vi "Wrap TPCANMessageType.vi"(10 "TPCANMessageType Numeric":u8) -> (2 "TPCANMessageType out Strings":string, 3 "TPCANMessageType Numeric out":u8)   [LabVIEW 2016]
doc: "TPCANMessageType defines the Message type\nof a CAN message that should be send.\nIn the case of seinding a CAN message\nit can have the values below.\n\nPCAN Message Types:\nPCAN_MESSAGE_STANDARD 0x00\nPCAN_MESSAGE_RTR 0x01\nPCAN_MESSAGE_EXTENDED 0x02\nPCAN_MESSAGE_FD 0x04\nPCAN_MESSAGE_BRS 0x08\nPCAN_MESSAGE_ESI 0x10\nPCAN_MESSAGE_STATUS 0x80\n\nIn case of receiving messages from the\nPCAN driver is can look like the the list \nbefore but it also can be a bitfild.\nThat means that more than exact one\nreturn value within a single numeric is\npossible.\nTo make things more easy the VI is\ncapable to decode the PCAN drivers\nreturned value."
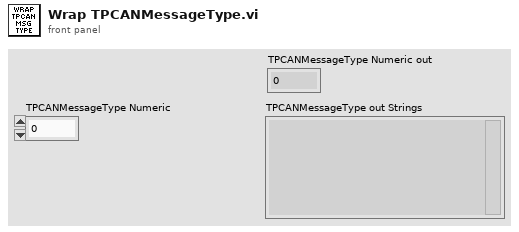
[diagram p1: front panel]
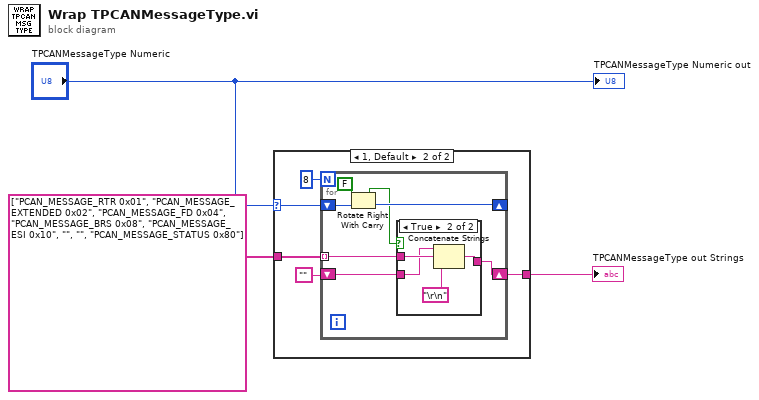
[diagram p0: block diagram]
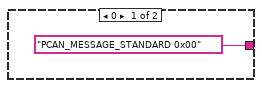
[diagram p2: hidden frame]
diagram:
  n1 = case shown="1, Default" "TPCANMessageType Numeric" {
    selector: "TPCANMessageType Numeric" -> [_ w5]
    tunnel: string[] ["PCAN_MESSAGE_RTR 0x01", "PCAN_MESSAGE_EXTENDED 0x02", "PCAN_MESSAGE_FD 0x04", "PCAN_MESSAGE_BRS 0x08", "PCAN_MESSAGE_ESI 0x10", "", "", "PCAN_MESSAGE_STATUS 0x80"] ("appended array") -> [_ w8]
    tunnel: ["PCAN_MESSAGE_STANDARD 0x00" w6] -> w1
    frame 0 {
    }
    frame 1, Default {
      n2 = for {
        N: 8 -> [_]
        shift-right: [w15] -> _
        shift-left: w5 -> [w16]
        tunnel: w8 -> [w12] mode=indexing
        shift-right: [w11] -> w6
        shift-left: "" -> [w10]
        n3 = Rotate Right With Carry(2:w16, 3:FALSE ("carry")) -> (0:w15:u8, 1:w13:bool)
        n4 = case shown="True" w13 {
          tunnel: w12 -> [_ w21]
          tunnel: [w17 w19] -> w11
          tunnel: w10 -> [w17 w18]
          frame False {
          }
          frame True {
            n5 = Concatenate Strings(w18, w21, "\r\n") -> (w19:string)
          }
        }
      }
    }
  }
  "TPCANMessageType out Strings" <- w1
  "TPCANMessageType Numeric out" <- "TPCANMessageType Numeric"
